vi "Create DI Task.vi"(8 "error in (no error)":errorcluster, 11 "DI Channel Setting":T1) -> (0 "error out":errorcluster, 3 "DI_Task":refnum<k21>)   [LabVIEW 2021, in "DAQ IO.lvlib"]
uses:
  DAQ IO.lvlib
  <vilib>/DAQmx/create/channels.llb/DAQmx Create Channel (DI-Digital Input).vi
  DI Channel Setting.ctl
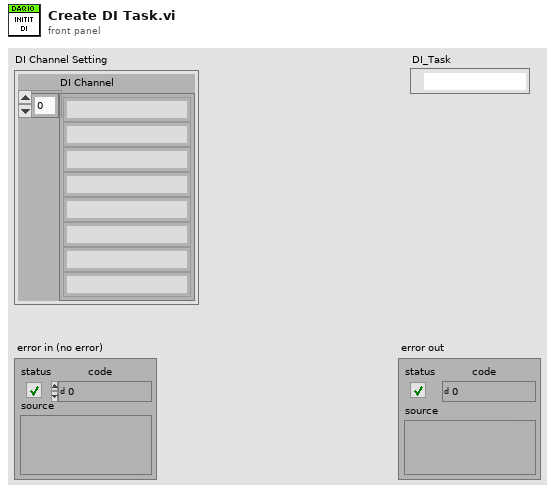
[diagram p1: front panel]
types:
  T1 = typedef "DAQ IO.lvlib/DI Channel Setting.ctl" = cluster{"DI Channel":string[]}
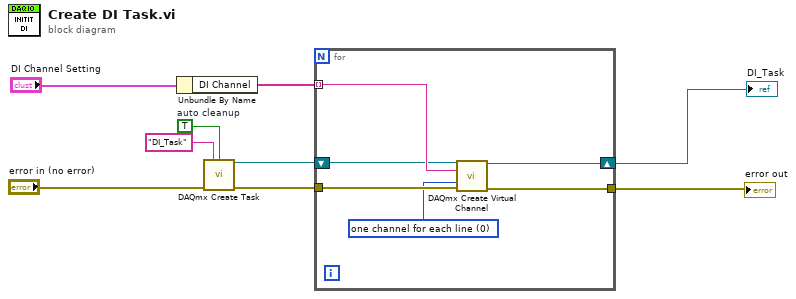
[diagram p0: block diagram]
diagram:
  w7 = TRUE  # auto cleanup
  n1 = Unbundle By Name("DI Channel Setting") -> ("DI Channel"=w6:string[])
  n2 = call <vilib>:"DAQmx Create Task.vi"("new task name"="DI_Task", "auto cleanup"=w7, "error in"="error in (no error)") -> ("task out"=w4:refnum<k21>, "error out"=w8:errorcluster)  [unwired: 11 in]
  n3 = for {
    tunnel: w8 -> [w15]
    tunnel: w6 -> [w13] mode=indexing
    tunnel: [w12] -> w5
    shift-right: [w10] -> w3
    shift-left: w4 -> [w11]
    w14 = 0 items=["one channel for each line", "one channel for all lines"] ("line grouping")
    n4 = call-poly <vilib>:"DAQmx Create Virtual Channel.vi"("task in"=w11, "lines"=w13, "line grouping"=w14, "error in"=w15) -> ("task out"=w10:refnum<k21>, "error out"=w12:errorcluster)  [unwired: 10 in]
  }
  "error out" <- w5
  "DI_Task" <- w3
